vi "_DServerRequestDataToDevStateArray.vi"(1 "value_in":u8[](array[numeric]), 2 "dim_y":i32, 3 "dim_x":i32) -> (0 "attribute value":T1=enum."UNKNOWN")   [LabVIEW 2014, in "tango.lvlib"]
uses:
  tango.lvlib
  Common VIs/Typedefs/_TangoState_t.ctl
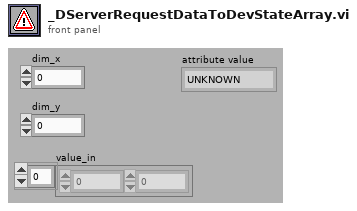
[diagram p1: front panel]
types:
  T1 = typedef "tango.lvlib/_TangoState_t.ctl" = enum32{"ON", "OFF", "CLOSE", "OPEN", "INSERT", "EXTRACT", "MOVING", "STANDBY", "FAULT", "INIT", "RUNNING", "ALARM", "DISABLE", "UNKNOWN"}
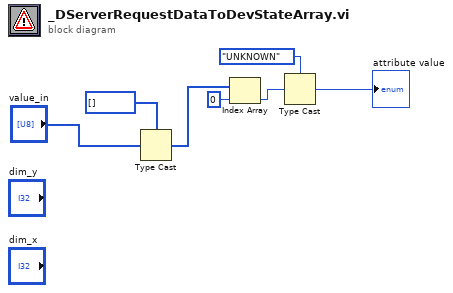
[diagram p0: block diagram]
diagram:
  n1 = Type Cast(type=u32[] [], x="value_in") -> (*(type *) &x=w5:u32[])
  n2 = Index Array(array=w5, index=0) -> (element=w3:u32)
  n3 = Type Cast(type=_TangoState_t."UNKNOWN" ("Tango Device State"), x=w3) -> (*(type *) &x=→"attribute value":T1)
